vi "API_DB.SelectRecord.vi"(6 "Timeout (ms)":u32, 7 "Wait (F)":bool, 8 "error in (no error)":errorcluster, 10 "QueryBuilderData":T1, 11 "Database in":refnum<class "Database.lvclass">) -> (0 "error out":errorcluster, 2 "Records":string[][](array[string]), 3 "Database out":refnum<class "Database.lvclass">)   [LabVIEW 2022 SP3, in "Database.lvclass"]
doc: "Developed by Kevin Thompson\nkevin@thompsonengineering.net\n\nCopyright 2018\nThompson Engineering, LLC"
uses:
  Database.lvclass
  DataTypes/QuiryBuilderData--Cluster.ctl
  DataTypes/AsynCmd_Temp01--enum.ctl
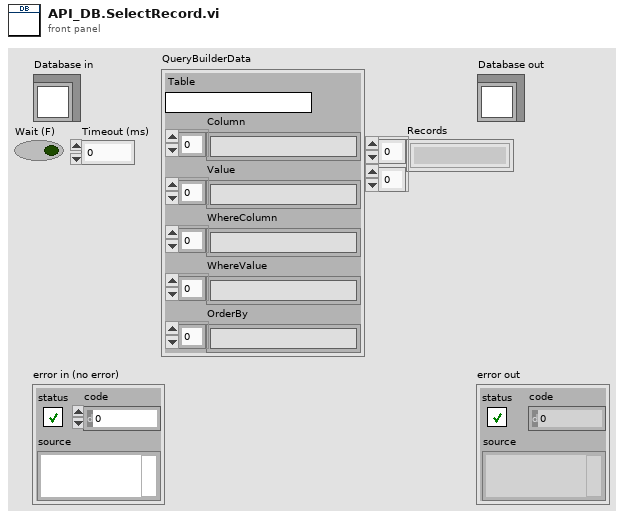
[diagram p1: front panel]
types:
  T1 = typedef "QuiryBuilderData--Cluster.ctl" = cluster{"Table":string, "Column":string[], "Value":string[], "WhereColumn":string[], "WhereValue":string[], "OrderBy":string[]}
  T2 = typedef "Database.lvclass/AsynCmd_Temp01--enum.ctl" = enum16{"DB.DeleteRecord", "DB.UpdateRecord", "DB.InsertRecord", "DB.SelectRecord", "DB.ExecuteSQLCommand", "DB.FindFirstSlot", "DB.GenericSQLQuery"}
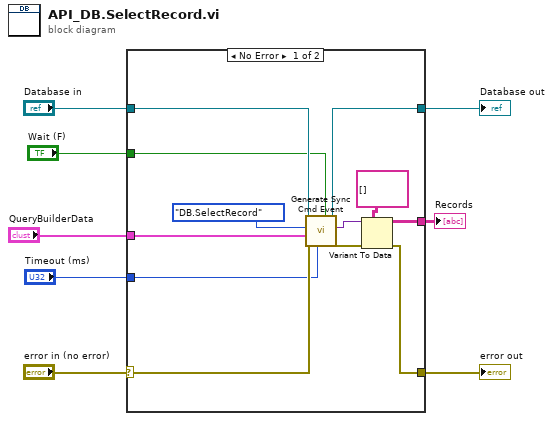
[diagram p0: block diagram]
diagram:
  n1 = case shown="No Error" "error in (no error)" {
    selector: "error in (no error)" -> [w18 w22]
    tunnel: [w11 w22] -> w7
    tunnel: [w19 w21] -> w5
    tunnel: "Database in" -> [w20 w21]
    tunnel: "QueryBuilderData" -> [w16 _]
    tunnel: [w13 _] -> w3
    tunnel: "Wait (F)" -> [w10 _]
    tunnel: "Timeout (ms)" -> [w9 _]
    frame No Error {
      n2 = call "Generate Sync Cmd Event.vi"("Wait (F)"=w10, "Timeout (ms)"=w9, "error in (no error)"=w18, "vData"=w16, "AsyncCmd"=AsynCmd_Temp01--enum."DB.SelectRecord", "Database in"=w20) -> ("error out"=w12:errorcluster, "Return Value"=w15:variant, "Database out"=w19:refnum<class "Database.lvclass">)  [unwired: 3 in]
      n3 = Variant To Data(error in=w12, type=string[][] [], Variant=w15) -> (data=w13:string[][], error out=w11:errorcluster)
    }
    frame Error {
    }
  }
  "error out" <- w7
  "Database out" <- w5
  "Records" <- w3
